vi "HEWH RLT PRAT.vi"() -> ()   [LabVIEW 2023] (continued)
        n1520 = call-poly "Enqueue Message.vi"("Priority Message? (F)"=TRUE, "Message"="Reset_Totalizer_UI", "Message Queue"=w3738) -> ("error out"=w3740:errorcluster, "dup Message Queue"=w3739:refnum<queue>)  [unwired: 7 in]
      }
      event "Reset Power Analyzer", "Start/Pause test": Value Change {
        n1521 = event-data() -> ()  [unwired: 1 in, 1 out]
        n1522 = call-poly "Enqueue Message.vi"("Priority Message? (F)"=TRUE, "Message"="Reset_PowerAnalyzer_UI", "Message Queue"=w3743) -> ("error out"=w3745:errorcluster, "dup Message Queue"=w3744:refnum<queue>)  [unwired: 7 in]
      }
      event "Manual Heating Value": Value Change {
        n1523 = event-data() -> ("NewVal"=w3748:bool)  [unwired: 1 in, 2 out]
        n1524 = call-poly "Enqueue Message.vi"("Priority Message? (F)"=TRUE, "Message Data"=w3748, "Message"="Manual_Heating_Value_UI", "Message Queue"=w3749) -> ("error out"=w3751:errorcluster, "dup Message Queue"=w3750:refnum<queue>)  [unwired: 6 in]
      }
      event "HHV-LP-Manual": Value Change {
        n1525 = event-data() -> ("NewVal"=w3754:sgl)  [unwired: 1 in, 2 out]
        n1526 = call-poly "Enqueue Message.vi"("Priority Message? (F)"=TRUE, "Message Data"=w3754, "Message"="Heating_Value_Adjust_LP_UI", "Message Queue"=w3755) -> ("error out"=w3757:errorcluster, "dup Message Queue"=w3756:refnum<queue>)  [unwired: 6 in]
      }
      event "HHV-NG-Manual": Value Change {
        n1527 = event-data() -> ("NewVal"=w3760:sgl)  [unwired: 1 in, 2 out]
        n1528 = call-poly "Enqueue Message.vi"("Priority Message? (F)"=TRUE, "Message Data"=w3760, "Message"="Heating_Value_Adjust_NG_UI", "Message Queue"=w3761) -> ("error out"=w3763:errorcluster, "dup Message Queue"=w3762:refnum<queue>)  [unwired: 6 in]
      }
      event "Update Vesta Temp": Value Change {
        n1529 = event-data() -> ()  [unwired: 1 in, 3 out]
        n1530 = call-poly "Enqueue Message.vi"("Priority Message? (F)"=TRUE, "Message Data"="Temperature Parameters", "Message"="PUT_Vesta_Temp_UI", "Message Queue"=w3768) -> ("dup Message Queue"=w3767:refnum<queue>)  [unwired: 6 in, 1 out]
      }
      event "Update Enviracom Status": Value Change {
        n1531 = event-data() -> ()  [unwired: 1 in, 1 out]
        n1532 = case shown="\"Burner OFF\", Default" "Burner Status" {
          tunnel: [FALSE TRUE] -> w3771
          frame "Burner OFF", Default {
          }
          frame "Burner ON" {
          }
        }
        n1533 = call-poly "Enqueue Message.vi"("Priority Message? (F)"=TRUE, "Message Data"=w3771, "Message"="PUT_EnviraCom_Temp_UI", "Message Queue"=w3775) -> ("error out"=w3773:errorcluster, "dup Message Queue"=w3774:refnum<queue>)  [unwired: 6 in]
      }
      event "Vesta COM Port": Value Change {
        n1534 = event-data() -> ("NewVal"=w3781:refnum<visa-resource-name>)  [unwired: 1 in]
        n1535 = property class="Instr"(reference=w3781) -> ("Rsrc Name"=w3780:string)  [unwired: 1 in, 2 out]
        n1536 = call-poly "Enqueue Message.vi"("Priority Message? (F)"=TRUE, "Message Data"=w3780, "Message"="Set_Vesta_VISA_Name_UI", "Message Queue"=w3784) -> ("error out"=w3782:errorcluster, "dup Message Queue"=w3783:refnum<queue>)  [unwired: 6 in]
      }
      event "Ultramat  COM Port": Value Change {
        n1537 = event-data() -> ("NewVal"=w3788:refnum<visa-resource-name>)  [unwired: 1 in]
        n1538 = property class="Serial Instr"(reference=w3788) -> ("Rsrc Name"=w3787:string)  [unwired: 1 in, 2 out]
        n1539 = call-poly "Enqueue Message.vi"("Priority Message? (F)"=TRUE, "Message Data"=w3787, "Message"="Set_Ultramat_VISA_Name_UI", "Message Queue"=w3791) -> ("error out"=w3789:errorcluster, "dup Message Queue"=w3790:refnum<queue>)  [unwired: 6 in]
      }
      event "MW100 COM Port": Value Change {
        n1540 = event-data() -> ("NewVal"=w3795:refnum<visa-resource-name>)  [unwired: 1 in]
        n1541 = property class="Instr"(reference=w3795) -> ("Rsrc Name"=w3794:string)  [unwired: 1 in, 2 out]
        n1542 = call-poly "Enqueue Message.vi"("Priority Message? (F)"=TRUE, "Message Data"=w3794, "Message"="Set_MW100_VISA_Name_UI", "Message Queue"=w3798) -> ("error out"=w3796:errorcluster, "dup Message Queue"=w3797:refnum<queue>)  [unwired: 6 in]
      }
      event "Agilent COM Port": Value Change {
        n1543 = event-data() -> ("NewVal"=w3802:refnum<visa-resource-name>)  [unwired: 1 in]
        n1544 = property class="Instr"(reference=w3802) -> ("Rsrc Name"=w3801:string)  [unwired: 1 in, 2 out]
        n1545 = call-poly "Enqueue Message.vi"("Priority Message? (F)"=TRUE, "Message Data"=w3801, "Message"="Set_Agilent_VISA_Name_UI", "Message Queue"=w3805) -> ("error out"=w3803:errorcluster, "dup Message Queue"=w3804:refnum<queue>)  [unwired: 6 in]
      }
      event "Alicat COM Port": Value Change {
        n1546 = event-data() -> ("NewVal"=w3809:refnum<visa-resource-name>)  [unwired: 1 in]
        n1547 = property class="Instr"(reference=w3809) -> ("Rsrc Name"=w3808:string)  [unwired: 1 in, 2 out]
        n1548 = call-poly "Enqueue Message.vi"("Priority Message? (F)"=TRUE, "Message Data"=w3808, "Message"="Set_Alicat_VISA_Name_UI", "Message Queue"=w3812) -> ("error out"=w3810:errorcluster, "dup Message Queue"=w3811:refnum<queue>)  [unwired: 6 in]
      }
      event "Ritter COM Port": Value Change {
        n1549 = event-data() -> ("NewVal"=w3816:refnum<visa-resource-name>)  [unwired: 1 in]
        n1550 = property class="Instr"(reference=w3816) -> ("Rsrc Name"=w3815:string)  [unwired: 1 in, 2 out]
        n1551 = call-poly "Enqueue Message.vi"("Priority Message? (F)"=TRUE, "Message Data"=w3815, "Message"="Set_Ritter_VISA_Name_UI", "Message Queue"=w3819) -> ("error out"=w3817:errorcluster, "dup Message Queue"=w3818:refnum<queue>)  [unwired: 6 in]
      }
      event "Heise Barometer COM Port": Value Change {
        n1552 = event-data() -> ("NewVal"=w3823:refnum<visa-resource-name>)  [unwired: 1 in]
        n1553 = property class="Instr"(reference=w3823) -> ("Rsrc Name"=w3822:string)  [unwired: 1 in, 2 out]
        n1554 = call-poly "Enqueue Message.vi"("Priority Message? (F)"=TRUE, "Message Data"=w3822, "Message"="Set_Heise_VISA_Name_UI", "Message Queue"=w3826) -> ("error out"=w3824:errorcluster, "dup Message Queue"=w3825:refnum<queue>)  [unwired: 6 in]
      }
      event "WT300 COM Port": Value Change {
        n1555 = event-data() -> ("NewVal"=w3830:refnum<visa-resource-name>)  [unwired: 1 in]
        n1556 = property class="Instr"(reference=w3830) -> ("Rsrc Name"=w3829:string)  [unwired: 1 in, 2 out]
        n1557 = call-poly "Enqueue Message.vi"("Priority Message? (F)"=TRUE, "Message Data"=w3829, "Message"="Set_WT300_VISA_Name_UI", "Message Queue"=w3833) -> ("error out"=w3831:errorcluster, "dup Message Queue"=w3832:refnum<queue>)  [unwired: 6 in]
      }
      event "Laurel IP Address": Value Change {
        n1558 = event-data() -> ("NewVal"=w3836:string)  [unwired: 1 in]
        n1559 = call-poly "Enqueue Message.vi"("Priority Message? (F)"=TRUE, "Message Data"=w3836, "Message"="Set_Laurel_IP_Name_UI", "Message Queue"=w3839) -> ("error out"=w3837:errorcluster, "dup Message Queue"=w3838:refnum<queue>)  [unwired: 6 in]
      }
      event "Emerson IP Address": Value Change {
        n1560 = event-data() -> ("NewVal"=w3842:string)  [unwired: 1 in]
        n1561 = call-poly "Enqueue Message.vi"("Priority Message? (F)"=TRUE, "Message Data"=w3842, "Message"="Set_Emerson_IP_Name_UI", "Message Queue"=w3845) -> ("error out"=w3843:errorcluster, "dup Message Queue"=w3844:refnum<queue>)  [unwired: 6 in]
      }
      event "NG Inficon IP Address": Value Change {
        n1562 = event-data() -> ("NewVal"=w3848:string)  [unwired: 1 in]
        n1563 = call-poly "Enqueue Message.vi"("Priority Message? (F)"=TRUE, "Message Data"=w3848, "Message"="Set_NG_Inficon_IP_Name_UI", "Message Queue"=w3851) -> ("error out"=w3849:errorcluster, "dup Message Queue"=w3850:refnum<queue>)  [unwired: 6 in]
      }
      event "LP Inficon IP Address": Value Change {
        n1564 = event-data() -> ("NewVal"=w3854:string)  [unwired: 1 in]
        n1565 = call-poly "Enqueue Message.vi"("Priority Message? (F)"=TRUE, "Message Data"=w3854, "Message"="Set_LP_Inficon_IP_Name_UI", "Message Queue"=w3857) -> ("error out"=w3855:errorcluster, "dup Message Queue"=w3856:refnum<queue>)  [unwired: 6 in]
      }
      event "Viasala IP Address": Value Change {
        n1566 = event-data() -> ("NewVal"=w3860:string)  [unwired: 1 in]
        n1567 = call-poly "Enqueue Message.vi"("Priority Message? (F)"=TRUE, "Message Data"=w3860, "Message"="Set_Viasala_IP_Name_UI", "Message Queue"=w3863) -> ("error out"=w3861:errorcluster, "dup Message Queue"=w3862:refnum<queue>)  [unwired: 6 in]
      }
      event "Tenney IP Address": Value Change {
        n1568 = event-data() -> ("NewVal"=w3866:string)  [unwired: 1 in]
        n1569 = call-poly "Enqueue Message.vi"("Priority Message? (F)"=TRUE, "Message Data"=w3866, "Message"="Set_Tenney_IP_Name_UI", "Message Queue"=w3869) -> ("error out"=w3867:errorcluster, "dup Message Queue"=w3868:refnum<queue>)  [unwired: 6 in]
      }
      event Value Change {
        n1570 = event-data() -> ("NewVal"=w3872:T50)  [unwired: 1 in]
        n1571 = call-poly "Enqueue Message.vi"("Priority Message? (F)"=TRUE, "Message Data"=w3872, "Message"="Set_Agilent_Station_UI", "Message Queue"=w3875) -> ("error out"=w3873:errorcluster, "dup Message Queue"=w3874:refnum<queue>)  [unwired: 6 in]
      }
      event Value Change {
        n1572 = event-data() -> ("NewVal"=w3879:T49)  [unwired: 1 in]
        n1573 = call-poly "Enqueue Message.vi"("Priority Message? (F)"=TRUE, "Message Data"=w3879, "Message"="GEA3_StationA_Board_ID_UI", "Message Queue"=w3880) -> ("error out"=w3881:errorcluster, "dup Message Queue"=w3878:refnum<queue>)  [unwired: 6 in]
      }
      event Value Change {
        n1574 = event-data() -> ("NewVal"=w3885:T49)  [unwired: 1 in]
        n1575 = call-poly "Enqueue Message.vi"("Priority Message? (F)"=TRUE, "Message Data"=w3885, "Message"="GEA3_StationB_Board_ID_UI", "Message Queue"=w3886) -> ("error out"=w3887:errorcluster, "dup Message Queue"=w3884:refnum<queue>)  [unwired: 6 in]
      }
      event Value Change {
        n1576 = event-data() -> ("NewVal"=w3891:T49)  [unwired: 1 in]
        n1577 = call-poly "Enqueue Message.vi"("Priority Message? (F)"=TRUE, "Message Data"=w3891, "Message"="GEA3_StationC_Board_ID_UI", "Message Queue"=w3892) -> ("error out"=w3893:errorcluster, "dup Message Queue"=w3890:refnum<queue>)  [unwired: 6 in]
      }
      event Value Change {
        n1578 = event-data() -> ("NewVal"=w3897:T49)  [unwired: 1 in]
        n1579 = call-poly "Enqueue Message.vi"("Priority Message? (F)"=TRUE, "Message Data"=w3897, "Message"="GEA3_StationD_Board_ID_UI", "Message Queue"=w3898) -> ("error out"=w3899:errorcluster, "dup Message Queue"=w3896:refnum<queue>)  [unwired: 6 in]
      }
      event "Enviracom COM Port": Value Change {
        n1580 = event-data() -> ("NewVal"=w3903:refnum<visa-resource-name>)  [unwired: 1 in]
        n1581 = property class="Instr"(reference=w3903) -> ("Rsrc Name"=w3902:string)  [unwired: 1 in, 2 out]
        n1582 = call-poly "Enqueue Message.vi"("Priority Message? (F)"=TRUE, "Message Data"=w3902, "Message"="Set_Envira_VISA_Name_UI", "Message Queue"=w3906) -> ("error out"=w3904:errorcluster, "dup Message Queue"=w3905:refnum<queue>)  [unwired: 6 in]
      }
    }
    n1583 = call "Tenney Error Handler - Event Handling Loop.vi"("error in (no error)"=w3410, "Message Queue"=w3408) -> ("dup error in"=w3407:errorcluster)  [unwired: 8 in, 1 out]
  }
  n1584 = while {
    tunnel: w59 -> [w3937]
    shift-right: [w3943] -> _
    shift-left: T67 {"Timer Data"={"Station A-Timer"=[], "Station B-Timer"=[], "Station C-Timer"=[], "Station D-Timer"=[], "Timer A"=0.0, "Timer B"=0.0, "Timer C"=0.0, "Timer D"=0.0, "TimerA (String)"="", "TimerB (String)"="", "TimerC (String)"="", "TimerD (String)"="", "TimerA (H:M:S)"="", "TimerB (H:M:S)"="", "TimerC (H:M:S)"="", "TimerD (H:M:S)"=""}, "Tenney Data"={"Temperature Setpoint"=0.0, "Temperature Process Variable"=0.0, "Humidity Setpoint"=0.0, "Humidity Process Variable"=0.0, "Frequency Setpoint"=0.0, "Frequency Process Variable"=0.0, "Chamber Status (ON/OFF)"=""}, "Viasala Data Output"={"Temperature Probe 1"=0.0, "Humidity Probe 1"=0.0, "Temperature Probe 2"=0.0, "Humidity Probe 2"=0.0}, "Alicat Data"={"Data Cluster"={"Absolute Pressure"=0.0, "Gauge/Diff. Pressure"=0.0, "Barometric Pressure"=0.0, "Temperature"=0.0, "Volumetric Flow"=0.0, "Mass Flow"=0.0, "Setpoint"=0.0, "Valve Drive"=0.0, "Totalizer"=0.0, "[hr]"=0.0, "[min]"=0.0, "[sec]"=0.0, "Totalizer Average Flow"=0.0, "Totalizer Peak Flow"=0.0, "Gas selected"=""}, "Units of Measure Input"={"Abs. Pressure"="", "Gauge/Diff. Press."="", "Barometric Press."="", "Temperature"="", "Volume"="", "Mass"="", "Setpoint"="", "Valve Drive"="", "Totalizer"="", "Tot. Timer"="", "Tot. Avg. Flow"="", "Tot. Peak Flow"=""}, "Header Array"=[]}, "Inficon Data"={"Gross Heating Value, Vol (Real, Dry)"=0.0, "Nitrogen Component Normalized Mole % (Dry)"=0.0, "Methane Component Normalized Mole % (Dry)"=0.0, "Carbon Dioxide Component Normalized Mole % (Dry)"=0.0, "Ethane Component Normalized Mole % (Dry)"=0.0, "Propane Component Normalized Mole % (Dry)"=0.0, "i-Pentane Component Normalized Mole % (Dry)"=0.0, "i-Butane Component Normalized Mole % (Dry)"=0.0, "n-Butane Component Normalized Mole % (Dry)"=0.0, "n-Pentane Component Normalized Mole % (Dry)"=0.0, "Hexane Component Normalized Mole % (Dry)"=0.0, "Heptane Component Normalized Mole % (Dry)"=0.0, "Gross Wobbe Index, Real(Dry)"=0.0, "Relative Density, Real(Dry)"=0.0, "Propylene Component Normalized Mole % (Dry)"=0.0, "C4 Olefins Component Normalized Mole % (Dry)"=0.0, "Water Component Normalized Mole % (Dry)"=0.0, "Gross Heating Value, Vol (Real, Sat)"=0.0, "Natural Gas Data"=[], "Propane Data"=[]}, "Inficon Data LP"={"Gross Heating Value, Vol (Real, Dry)"=0.0, "Nitrogen Component Normalized Mole % (Dry)"=0.0, "Methane Component Normalized Mole % (Dry)"=0.0, "Carbon Dioxide Component Normalized Mole % (Dry)"=0.0, "Ethane Component Normalized Mole % (Dry)"=0.0, "Propane Component Normalized Mole % (Dry)"=0.0, "i-Pentane Component Normalized Mole % (Dry)"=0.0, "i-Butane Component Normalized Mole % (Dry)"=0.0, "n-Butane Component Normalized Mole % (Dry)"=0.0, "n-Pentane Component Normalized Mole % (Dry)"=0.0, "Hexane Component Normalized Mole % (Dry)"=0.0, "Heptane Component Normalized Mole % (Dry)"=0.0, "Gross Wobbe Index, Real(Dry)"=0.0, "Relative Density, Real(Dry)"=0.0, "Propylene Component Normalized Mole % (Dry)"=0.0, "C4 Olefins Component Normalized Mole % (Dry)"=0.0, "Water Component Normalized Mole % (Dry)"=0.0, "Gross Heating Value, Vol (Real, Sat)"=0.0, "Natural Gas Data"=[], "Propane Data"=[]}, "Ultramat 23 Data"=[], "Ritter Data"={"Gas Flow Rate (L/hr)-Uncorrected"=0.0, "Totalized Flow (L)--Uncorrected"=0.0, "Gas Flow Rate (cuft/hr)-Uncorrected"=0.0, "Totalized Flow (cuft)-Uncorrected"=0.0, "Gas Temperature (F)"=0.0, "Gas Pressure (in WC)"=0.0, "Heise Barometric Pressure (inHG)"=0.0, "STP Correction Factor"=0.0, "Temp Correction Factor"=0.0, "Pressure Correction Factor"=0.0, "Water Vapor Pressure"=0.0, "Gas Flow Rate (cuft/hr)-Corrected"=0.0, "Totalized Flow (cuft)-Corrected"=0.0, "Gas BTU"=0.0, "Gas BTU/hr"=0.0, "Gas Flow Rate (cuft/hr)-Uncorrected-Raw"=0.0}, "Heise Data"=0.0, "Emerson Data"={"Mass Flow Rate (Scaled Integer)"=0, "Density (Scaled Integer)"=0, "Temperature (Scaled Integer)"=0, "Volume Flow Rate (Scaled Integer)"=0, "Totalizer 1 (Scaled Integer)"=0, "Totalizer 2 (Scaled Integer)"=0, "Transmitter Software Rev"=0, "Flow Direction"="", "Mass Flow Units"="", "Density Units"="", "Temperature Units"="", "Volume Flow Units"="", "Pressure Units"="", "Mass Total Units"="", "Volume Total Units"="", "Inventory 1 (Scaled Integer)"=0, "Inventory 2 (Scaled Integer)"=0, "Mass Flow Rate"=0.0, "Density"=0.0, "Temperature"=0.0, "Volume Flow Rate"=0.0, "Pressure (Scaled Integer)"=0, "Current Value Totalizer 1 (Pounds per draw)"=0.0, "Current Value Totalizer 2 (Gallons per draw)"=0.0, "Current Value Inventory 1 (Pounds Total)"=0.0, "Current Value Inventory 2 (Gallons Total)"=0.0, "Drive Gain"=0.0, "Raw Tube Frequency (Hz)"=0.0, "Dynamic Viscosity (Centipoise)"=0.0, "Kinematic Viscosity (Centistokes)"=0.0, "Hot Gallons (Calculated Gallons)"=0.0, "Hot Flow Rate (Calculated GPM)"=0.0, "Hot Gallons Inventory (Gallons)"=0.0, "Hot Flow Rate (Laurel)"=0.0, "Hot Gallons (Laurel)"=0.0}, "Laurel Meter Data"={"Flow Rate (GPM)"=0.0, "Totalized Flow (Gallons)"=0.0}, "WT300 Data"={"Current (A):Element 1"=0.0, "Current (A):Element 2"=0.0, "Power (W):Sigma"=0.0, "Watt Hours (Wh):Sigma"=0.0, "Voltage (V):Element 2"=0.0, "Voltage (V):Element 1"=0.0, "Current Crest Factor:Element 1"=0.0, "Current Crest Factor:Element 2"=0.0, "Voltage Harmonic (%):Element 1"=0.0, "Voltage Harmonic (%):Element 2"=0.0, "Voltage Crest Factor:Element 1"=0.0, "Voltage Crest Factor:Element 2"=0.0, "Time:Element 1"=0.0, "Frequency (Hz):Element 1"=0.0, "Apparent Power (VA):Element 1"=0.0, "Apparent Power (VA):Element 2"=0.0, "Power Factor:Element 1"=0.0, "Power Factor:Element 2"=0.0, "Max Watt Hours"=0.0, "Voltage (V):Element 2 Avg"=0.0, "Voltage (V):Element 1 Avg"=0.0}, "Agilent Data"={"Location 11 (Channel 111)"=0.0, "Location 12 (Channel 112)"=0.0, "Location 13 (Channel 113)"=0.0, "Location 14 (Channel 114)"=0.0, "Location 15 (Channel 115)"=0.0, "Location 16 (Channel 116)"=0.0, "Location 17 (Channel 109)"=0.0, "Location 18 (Channel 110)"=0.0, "Location 19 (Channel 201)"=0.0, "Location 20 (Channel 202)"=0.0, "Location 21 (Channel 203)"=0.0, "Location 22 (Channel 204)"=0.0, "Location 23 (Channel 205)"=0.0, "Location 24 (Channel 206)"=0.0, "Location 25 (Channel 207)"=0.0, "Location 26 (Channel 208)"=0.0, "Location 27 (Channel 209)"=0.0, "Location 28 (Channel 210)"=0.0, "Location 29 (Channel 211)"=0.0, "Location 30 (Channel 212)"=0.0, "Location 31 (Channel 213)"=0.0, "Location 32 (Channel 214)"=0.0, "Location 33 (Channel 215)"=0.0, "Location 34 (Channel 216)"=0.0, "Location 35 (Channel 107)"=0.0, "Location 36 (Channel 108)"=0.0, "Location 37 (Channel 301)"=0.0, "Location 38 (Channel 302)"=0.0, "Location 39 (Channel 303)"=0.0, "Location 40 (Channel 304)"=0.0, "Location 41 (Channel 305)"=0.0, "Location 42 (Channel 306)"=0.0, "Location 43 (Channel 307)"=0.0, "Location 44 (Channel 308)"=0.0, "Location 45 (Channel 309)"=0.0, "Location 46 (Channel 310)"=0.0, "Location 47 (Channel 311)"=0.0, "Location 48 (Channel 312)"=0.0, "Location 49 (Channel 313)"=0.0, "Location 50 (Channel 314)"=0.0, "Location 51 (Channel 315)"=0.0, "Location 52 (Channel 316)"=0.0, "Location 53 (Channel 105)"=0.0, "Location 54 (Channel 106)"=0.0}, "GEA Data - Station A"={"ERD Data Input"={"Mixing Valve"={"T7 Temp (°F) - (0x40B9)"=0.0, "MixValveAbsoluteStepPosition - (0x400B)"=0, "Flow State - (0X4069)"=0, "T6 Temp (°F) - (0x406E)"=0.0}, "Standard ERDs"={"User UI Mode (0X4020)"="", "User Setpoint (0x4024)"=0, "Compressor (0x4068)"=FALSE, "Lower Element (0x4068)"=FALSE, "Upper Element (0x4068)"=FALSE, "Fan (0x4068)"=FALSE, "T1 Temp Lower Tank (°F) - (0x405F)"=0.0, "T2 Temp Upper Tank (°F) - (0x4060)"=0.0, "Line Voltage (0x4066)"=0, "MeasuredCurrent (0x4065)"=0.0, "Tank Setpoint (°F) - (0x4026)"=0, "Depletion - (0x40CB)"=0, "Personality - (0x0035)"=0}, "Heat Pump"={"EEV Position - (0X4067)"=0, "T3A TEMP EVAP IN (°F) - (0x4061)"=0.0, "T3B TEMP EVAP OUT (°F) -(0x4062)"=0.0, "T4 TEMP COMP DISCHARGE (°F) - (0x4063)"=0.0, "T5 TEMP AMBIENT (°F)- (0x4064)"=0.0, "Condensate Sensor - (0x40BC)"=0, "Fan (RPM) - (0xF073)"=0, "PWM (%) - (0xF056)"=0, "Compressor Speed (RPM) - (0xF093)"=0, "Compressor Target (RPM) - (0xF081)"=0, "Compressor Power (W) - (0xF092)"=0, "CPU Temperature (°F) - (0x40BA)"=0.0, "Board Temperature (°F) - (0x40BB)"=0.0}, "Inverter"={"Inverter IGBT Temp (°C) - (0xF280)"=0.0, "Inverter Chip Temp (°C) - (0xF284)"=0.0}}, "ERD Data"=[]}, "GEA Data - Station B"={"ERD Data Input"={"Mixing Valve"={"T7 Temp (°F) - (0x40B9)"=0.0, "MixValveAbsoluteStepPosition - (0x400B)"=0, "Flow State - (0X4069)"=0, "T6 Temp (°F) - (0x406E)"=0.0}, "Standard ERDs"={"User UI Mode (0X4020)"="", "User Setpoint (0x4024)"=0, "Compressor (0x4068)"=FALSE, "Lower Element (0x4068)"=FALSE, "Upper Element (0x4068)"=FALSE, "Fan (0x4068)"=FALSE, "T1 Temp Lower Tank (°F) - (0x405F)"=0.0, "T2 Temp Upper Tank (°F) - (0x4060)"=0.0, "Line Voltage (0x4066)"=0, "MeasuredCurrent (0x4065)"=0.0, "Tank Setpoint (°F) - (0x4026)"=0, "Depletion - (0x40CB)"=0, "Personality - (0x0035)"=0}, "Heat Pump"={"EEV Position - (0X4067)"=0, "T3A TEMP EVAP IN (°F) - (0x4061)"=0.0, "T3B TEMP EVAP OUT (°F) -(0x4062)"=0.0, "T4 TEMP COMP DISCHARGE (°F) - (0x4063)"=0.0, "T5 TEMP AMBIENT (°F)- (0x4064)"=0.0, "Condensate Sensor - (0x40BC)"=0, "Fan (RPM) - (0xF073)"=0, "PWM (%) - (0xF056)"=0, "Compressor Speed (RPM) - (0xF093)"=0, "Compressor Target (RPM) - (0xF081)"=0, "Compressor Power (W) - (0xF092)"=0, "CPU Temperature (°F) - (0x40BA)"=0.0, "Board Temperature (°F) - (0x40BB)"=0.0}, "Inverter"={"Inverter IGBT Temp (°C) - (0xF280)"=0.0, "Inverter Chip Temp (°C) - (0xF284)"=0.0}}, "ERD Data"=[]}, "GEA Data - Station C"={"ERD Data Input"={"Mixing Valve"={"T7 Temp (°F) - (0x40B9)"=0.0, "MixValveAbsoluteStepPosition - (0x400B)"=0, "Flow State - (0X4069)"=0, "T6 Temp (°F) - (0x406E)"=0.0}, "Standard ERDs"={"User UI Mode (0X4020)"="", "User Setpoint (0x4024)"=0, "Compressor (0x4068)"=FALSE, "Lower Element (0x4068)"=FALSE, "Upper Element (0x4068)"=FALSE, "Fan (0x4068)"=FALSE, "T1 Temp Lower Tank (°F) - (0x405F)"=0.0, "T2 Temp Upper Tank (°F) - (0x4060)"=0.0, "Line Voltage (0x4066)"=0, "MeasuredCurrent (0x4065)"=0.0, "Tank Setpoint (°F) - (0x4026)"=0, "Depletion - (0x40CB)"=0, "Personality - (0x0035)"=0}, "Heat Pump"={"EEV Position - (0X4067)"=0, "T3A TEMP EVAP IN (°F) - (0x4061)"=0.0, "T3B TEMP EVAP OUT (°F) -(0x4062)"=0.0, "T4 TEMP COMP DISCHARGE (°F) - (0x4063)"=0.0, "T5 TEMP AMBIENT (°F)- (0x4064)"=0.0, "Condensate Sensor - (0x40BC)"=0, "Fan (RPM) - (0xF073)"=0, "PWM (%) - (0xF056)"=0, "Compressor Speed (RPM) - (0xF093)"=0, "Compressor Target (RPM) - (0xF081)"=0, "Compressor Power (W) - (0xF092)"=0, "CPU Temperature (°F) - (0x40BA)"=0.0, "Board Temperature (°F) - (0x40BB)"=0.0}, "Inverter"={"Inverter IGBT Temp (°C) - (0xF280)"=0.0, "Inverter Chip Temp (°C) - (0xF284)"=0.0}}, "ERD Data"=[]}, "GEA Data - Station D"={"ERD Data Input"={"Mixing Valve"={"T7 Temp (°F) - (0x40B9)"=0.0, "MixValveAbsoluteStepPosition - (0x400B)"=0, "Flow State - (0X4069)"=0, "T6 Temp (°F) - (0x406E)"=0.0}, "Standard ERDs"={"User UI Mode (0X4020)"="", "User Setpoint (0x4024)"=0, "Compressor (0x4068)"=FALSE, "Lower Element (0x4068)"=FALSE, "Upper Element (0x4068)"=FALSE, "Fan (0x4068)"=FALSE, "T1 Temp Lower Tank (°F) - (0x405F)"=0.0, "T2 Temp Upper Tank (°F) - (0x4060)"=0.0, "Line Voltage (0x4066)"=0, "MeasuredCurrent (0x4065)"=0.0, "Tank Setpoint (°F) - (0x4026)"=0, "Depletion - (0x40CB)"=0, "Personality - (0x0035)"=0}, "Heat Pump"={"EEV Position - (0X4067)"=0, "T3A TEMP EVAP IN (°F) - (0x4061)"=0.0, "T3B TEMP EVAP OUT (°F) -(0x4062)"=0.0, "T4 TEMP COMP DISCHARGE (°F) - (0x4063)"=0.0, "T5 TEMP AMBIENT (°F)- (0x4064)"=0.0, "Condensate Sensor - (0x40BC)"=0, "Fan (RPM) - (0xF073)"=0, "PWM (%) - (0xF056)"=0, "Compressor Speed (RPM) - (0xF093)"=0, "Compressor Target (RPM) - (0xF081)"=0, "Compressor Power (W) - (0xF092)"=0, "CPU Temperature (°F) - (0x40BA)"=0.0, "Board Temperature (°F) - (0x40BB)"=0.0}, "Inverter"={"Inverter IGBT Temp (°C) - (0xF280)"=0.0, "Inverter Chip Temp (°C) - (0xF284)"=0.0}}, "ERD Data"=[]}, "MW100 Data"={"TC1-Channel 021"=0.0, "TC2-Channel 022"=0.0, "TC3-Channel 023"=0.0, "TC4-Channel 024"=0.0, "TC5-Channel 025"=0.0, "TC6-Channel 026"=0.0, "TC7-Channel 017"=0.0, "TC8-Channel 028"=0.0, "TC9-Channel 029"=0.0, "TC10-Channel 030"=0.0, "TC Tree Average"=0.0, "TC DWN- Channel 027"=0.0, "RTDin-Channel 031"=0.0, "RTDout-Channel 032"=0.0, "RTDamb-Channel 033"=0.0, "PSI1-Channel 011"=0.0, "PSI2-Channel 012"=0.0, "PSI3-Channel 013"=0.0, "PSI4-Channel 014"=0.0, "UE State-Channel 015"=0.0, "LE State-Channel 016"=0.0, "Module 4 Relay Status Output"={"INTELLIFAUCET TEMP(T)/FLOW(F) (CH 041)"=FALSE, "INTELLIFAUCET READY (CH 042)"=FALSE, "INTELLIFAUCET START (CH 043)"=FALSE, "INTELLIFAUCET STOP (CH 044)"=FALSE, "MAIN POWER RELAY (CH 047)"=FALSE, "NOT USED (CH 045)"=FALSE, "NOT USED (CH 046)"=FALSE, "PURGE VALVE RELAY (CH 048)"=FALSE, "OUTLET VALVE RELAY (CH 049)"=FALSE, "INLET VALVE RELAY (CH 050)"=FALSE, "Intellifaucet (% Open)"=0.0, "Proportioning Valve (%Open)"=0.0, "Intellifaucet Temp Setpoint (F)"=0.0}}, "Vesta Data Output"={"Temp_W_Raw_U"=0, "Temp_W_Raw_L"=0, "Temperature Water (F)"=0.0, "Temperature Water Compensated (F)"=0.0, "Temperature Ambient (F)"=0.0, "Setpoint Location (F)"=0.0, "Heat Request"="", "Fault Ram"="", "PWM DCDC Value"=0, "Pilot Voltage (mV)"=0.0, "Setpoint Actual (F)"=0.0, "Differential Actual (F)"=0.0, "Setpoint User (F)"=0.0, "Differential User (F)"=0.0, "Termperature FIltered -TCO (F)"=0.0, "Temp_C_Raw_1 - Sensor Voltage"="", "Temp_C_Raw_2 - Sensor Voltage"="", "Chamber Sensor Temperature (F)"=0.0, "LDO Base Temperature (F)"=0.0, "LDO Timer (sec)"=0, "Disabled (0)"=FALSE, "Warming (1)"=FALSE, "Heating (2)"=FALSE, "Cooling Data Write (3)"=FALSE, "Cooling (4)"=FALSE, "Data Read (5)"=FALSE, "N/A"=FALSE, "Temperature Trip (7)"=FALSE, "Burner"=FALSE}} ("Data Cluster") -> [w3944]
    tunnel: w68 -> [w3941]
    tunnel: w69 -> [w3940]
    tunnel: [w3935] -> w58
    tunnel: w72 -> [w3933]
    shift-right: [w3931] -> _
    shift-left: string[] [] -> [w3932]
    tunnel: w76 -> [w3929]
    tunnel: w55 -> [w3927]
    tunnel: w49 -> [w3926]
    tunnel: w48 -> [w3925]
    tunnel: w45 -> [w3924]
    tunnel: w43 -> [w3923]
    tunnel: w40 -> [w3922]
    tunnel: w35 -> [w3921]
    tunnel: w29 -> [w3920]
    tunnel: w28 -> [w3919]
    tunnel: w27 -> [w3918]
    tunnel: w26 -> [w3917]
    tunnel: w25 -> [w3916]
    tunnel: w24 -> [w3915]
    tunnel: w23 -> [w3914]
    tunnel: w22 -> [w3913]
    tunnel: w21 -> [w3912]
    tunnel: w20 -> [w3911]
    tunnel: w19 -> [w3910]
    tunnel: w18 -> [w3909]
    stop <- w3942 stop-if-true
    # "Message Handling Loop"
    n1585 = call "Dequeue Message.vi"("error in (no error)"=w3940, "Message Queue"=w3937) -> ("error out"=w3939:errorcluster, "Message Data"=w3938:variant, "Message"=w3930:string, "dup Message Queue"=w3936:refnum<queue>)  [unwired: 6 in]
    n1586 = case "Message Cases" shown="\"Process_Data\"" w3930 {
      selector: w3930 -> [_ w3952 _ _ _ _ _ _ _ _ _ _ _ _ _ _ _ _ _ _ _ _ _ _ _ _ _ _ _ _ _ _ _ _ _ _ _ _ _ _ _ _ _ _ _ _ _ _ _ _ _ _ _ _ _ _ _ _ _ _ _ _ _ _ _ _ _ _ _ _ _ _ _ _ _ _ _ _ _ _ _ _ _ _ _ _ _ _ _ _ _ _ _ _ _ _ _ _ _ _ _ _ _ _ _ _ _ _ _ _ _ _ _ _ _ _ _ _ _ _ _ _ _ _ _ _ _ _ _ _]
      tunnel: w3936 -> [_ _ w3970 _ w3996 _ _ _ _ _ _ _ w4030 _ _ _ _ _ _ _ _ _ _ _ _ _ _ _ _ _ _ _ _ _ _ _ _ w4205 _ _ _ _ _ _ _ _ w4281 _ _ _ _ _ _ _ _ _ _ _ _ w4386 _ _ w4409 _ _ w4432 _ _ w4455 _ _ w4478 _ _ _ _ _ _ _ _ _ _ _ _ _ _ w4606 _ _ _ w4638 _ _ w4661 _ _ _ _ w4700 _ _ _ w4729 _ _ _ _ w4773 _ _ _ w4806 _ _ _ w4841 _ _ _ _ _ w4884 _ _ _ w4915 _ _ _ w4948]
      tunnel: w3939 -> [w3951 _ w3969 w3977 w3990 w3999 w4003 w4004 w4011 w4017 w4023 w4029 w4039 w4040 w4048 w4058 w4065 w4072 w4079 w4086 w4093 w4100 w4107 w4114 w4121 w4128 w4135 w4142 w4149 w4156 w4163 w4170 w4176 w4182 w4189 w4196 w4203 w4213 w4215 w4223 w4231 w4243 w4251 w4259 w4266 w4274 w4290 w4292 w4300 w4306 w4314 w4322 w4330 w4338 w4345 w4353 w4361 w4369 w4379 w4395 w4397 w4405 w4418 w4420 w4428 w4441 w4443 w4451 w4464 w4466 w4474 w4487 w4489 w4492 w4505 w4517 w4529 w4541 w4559 w4560 w4572 w4579 w4586 w4588 w4596 w4605 w4615 w4617 w4625 w4637 w4647 w4649 w4657 w4670 w4672 w4680 w4689 w4699 w4709 w4711 w4719 w4724 w4738 w4740 w4748 w4757 w4769 w4782 w4784 w4792 w4802 w4815 w4817 w4825 w4835 w4848 w4850 w4858 w4868 w4872 w4880 w4893 w4895 w4903 w4909 w4924 w4926 w4934 w4944 w4957]
      tunnel: [w3949 w3953 w3966 w3971 w3993 w3997 w4002 w4004 w4007 w4013 w4019 w4025 w4031 w4040 w4045 w4054 w4061 w4068 w4075 w4082 w4089 w4096 w4103 w4110 w4117 w4124 w4131 w4138 w4145 w4152 w4159 w4166 w4172 w4178 w4185 w4192 w4199 w4214 w4215 w4220 w4236 w4244 w4252 w4260 w4271 w4279 w4291 w4292 w4297 w4310 w4318 w4326 w4334 w4342 w4349 w4357 w4365 w4373 w4376 w4396 w4397 w4402 w4419 w4420 w4425 w4442 w4443 w4448 w4465 w4466 w4471 w4488 w4489 w4491 w4502 w4515 w4527 w4539 w4552 w4560 w4572 w4579 w4586 w4588 w4593 w4600 w4616 w4617 w4622 w4634 w4648 w4649 w4654 w4671 w4672 w4677 w4685 w4691 w4710 w4711 w4716 w4725 w4739 w4740 w4745 w4760 w4765 w4783 w4784 w4789 w4798 w4816 w4817 w4822 w4831 w4849 w4850 w4854 w4864 w4872 w4877 w4894 w4895 w4900 w4913 w4925 w4926 w4931 w4941 w4958] -> w3934
      tunnel: w3944 -> [w3950 w3954 w3962 w3976 w3995 w3998 w4001 w4005 w4008 w4014 w4020 w4026 w4036 w4041 w4051 w4055 w4062 w4069 w4076 w4083 w4090 w4097 w4104 w4111 w4118 w4125 w4132 w4139 w4146 w4153 w4160 w4167 w4173 w4179 w4186 w4193 w4200 w4211 w4216 w4226 w4237 w4245 w4253 w4261 w4272 w4280 w4287 w4293 w4303 w4311 w4319 w4327 w4335 w4343 w4350 w4358 w4366 w4374 w4381 w4392 w4398 w4408 w4415 w4421 w4431 w4438 w4444 w4454 w4461 w4467 w4477 w4484 w4490 w4494 w4507 w4519 w4531 w4543 w4556 w4566 w4573 w4580 w4587 w4589 w4599 w4602 w4612 w4618 w4628 w4631 w4644 w4650 w4660 w4667 w4673 w4683 w4686 w4696 w4706 w4712 w4722 w4728 w4735 w4741 w4751 w4762 w4772 w4779 w4785 w4795 w4805 w4812 w4818 w4828 w4838 w4846 w4851 w4861 w4871 w4873 w4883 w4890 w4896 w4906 w4914 w4921 w4927 w4937 w4947 w4954]
      tunnel: [w3950 w3954 w3962 w3976 w3995 w3998 w4001 w4005 w4008 w4014 w4020 w4026 w4035 w4041 w4051 w4055 w4062 w4069 w4076 w4083 w4090 w4097 w4104 w4111 w4118 w4125 w4132 w4139 w4146 w4153 w4160 w4167 w4173 w4179 w4186 w4193 w4200 w4210 w4216 w4226 w4237 w4245 w4253 w4261 w4272 w4280 w4286 w4293 w4303 w4311 w4319 w4327 w4335 w4343 w4350 w4358 w4366 w4374 w4381 w4391 w4398 w4408 w4414 w4421 w4431 w4437 w4444 w4454 w4460 w4467 w4477 w4483 w4490 w4494 w4507 w4519 w4531 w4543 w4556 w4566 w4573 w4580 w4587 w4589 w4599 w4602 w4611 w4618 w4628 w4631 w4643 w4650 w4660 w4666 w4673 w4683 w4686 w4696 w4705 w4712 w4722 w4728 w4734 w4741 w4751 w4762 w4772 w4778 w4785 w4795 w4805 w4811 w4818 w4828 w4838 w4845 w4851 w4861 w4871 w4873 w4883 w4889 w4896 w4906 w4914 w4920 w4927 w4937 w4947 w4953] -> w3943
      tunnel: [_ _ _ _ TRUE _ _ _ _ _ _ _ _ _ _ _ _ _ _ _ _ _ _ _ _ _ _ _ _ _ _ _ _ _ _ _ _ _ _ _ _ _ _ _ _ _ _ _ _ _ _ _ _ _ _ _ _ _ _ _ _ _ _ _ _ _ _ _ _ _ _ _ _ _ _ _ _ _ _ _ _ _ _ _ _ _ _ _ _ _ _ _ _ _ _ _ _ _ _ _ _ _ _ _ _ _ _ _ _ _ _ _ _ _ _ _ _ _ _ _ _ _ _ _ _ _ _ _ _ _] -> w3942
      tunnel: w3938 -> [_ _ _ w3975 w3987 _ _ _ _ _ _ _ w4038 _ w4046 _ _ _ _ _ _ _ _ _ _ _ _ _ _ _ _ _ _ _ _ _ _ w4212 _ w4221 w4229 _ _ _ w4264 _ w4289 _ w4298 _ _ _ _ _ _ _ _ _ w4375 w4394 _ w4403 w4417 _ w4426 w4440 _ w4449 w4463 _ w4472 w4486 _ _ w4501 w4513 w4525 w4537 _ _ _ _ _ _ w4594 _ w4614 _ w4623 _ w4646 _ w4655 w4669 _ w4678 _ _ w4708 _ w4717 _ w4737 _ w4746 w4755 w4767 w4781 _ w4790 w4800 w4814 _ w4823 w4833 w4847 _ w4856 w4866 _ w4878 w4892 _ w4901 _ w4923 _ w4932 w4942 w4956]
      tunnel: w3941 -> [_ _ _ _ w3992 _ _ _ _ _ _ _ _ _ _ _ _ _ _ _ _ _ _ _ _ _ _ _ _ _ _ _ _ _ _ _ _ _ _ _ _ _ _ _ _ _ _ _ _ _ _ _ _ _ _ _ _ _ _ _ _ _ _ _ _ _ _ _ _ _ _ _ _ _ _ _ _ _ _ _ _ _ _ _ _ _ _ _ _ _ _ _ _ _ _ _ _ _ _ _ _ _ _ _ _ _ _ _ _ _ _ _ _ _ _ _ _ _ _ _ _ _ _ _ _ _ _ _ _ _]
      tunnel: w3933 -> [_ _ _ _ w3985 _ _ _ _ _ _ _ _ _ _ _ _ _ _ _ _ _ _ _ _ _ _ _ _ _ _ _ _ _ _ _ _ _ _ w4217 w4233 w4240 w4248 w4256 w4268 w4276 _ _ _ _ _ _ _ _ _ _ _ _ _ _ _ _ _ _ _ _ _ _ _ _ _ _ _ _ _ _ _ _ _ _ _ _ _ _ _ _ _ _ _ _ _ _ _ _ _ _ _ _ _ _ _ _ _ _ _ _ _ _ _ _ _ _ _ _ _ _ _ _ _ _ _ _ _ _ _ _ _ _ _ _]
      tunnel: w3929 -> [_ _ _ _ w3983 _ _ _ _ _ _ _ _ _ _ _ _ _ _ _ _ _ _ _ _ _ _ _ _ _ _ _ _ _ _ _ _ _ _ _ _ _ _ _ _ _ _ _ _ _ _ _ _ _ _ _ _ _ _ _ _ _ _ _ _ _ _ _ _ _ _ _ _ _ _ _ _ _ _ _ _ _ _ _ _ _ _ _ _ _ _ _ _ _ _ _ _ _ _ _ _ _ _ _ _ _ _ _ _ _ _ _ _ _ _ _ _ _ _ _ _ _ _ w4897 w4907 _ _ _ _ _]
      tunnel: w3927 -> [_ _ _ _ w3979 _ _ _ _ _ _ _ _ _ _ _ _ _ _ _ _ _ _ _ _ _ _ _ _ _ _ _ _ _ _ _ _ _ _ _ _ _ _ _ _ _ _ _ _ _ _ _ _ _ _ _ _ _ _ _ _ _ _ _ _ _ _ _ _ _ _ _ _ _ _ _ _ _ w4555 _ _ _ _ _ w4590 w4601 _ _ _ w4630 _ _ _ _ _ _ _ _ _ _ _ _ _ _ _ _ _ _ _ _ _ _ _ _ _ _ _ _ _ _ _ _ _ _ _ _ _ _ _ _]
      tunnel: w3926 -> [_ _ _ _ _ _ _ _ _ _ _ _ _ _ _ _ _ _ _ _ _ _ _ _ _ _ _ _ _ _ _ _ _ _ _ _ _ _ _ _ _ _ _ _ _ _ _ _ _ _ _ _ _ _ _ _ _ _ _ _ _ _ _ _ _ _ _ _ _ _ _ _ _ _ _ _ _ _ _ _ _ _ _ _ _ _ _ _ w4619 w4629 _ _ _ _ _ _ _ _ _ _ _ _ _ _ _ _ _ _ _ _ _ _ _ _ _ _ _ _ _ _ _ _ _ _ _ _ _ _ _ _]
      tunnel: w3925 -> [_ _ _ _ _ _ _ _ _ _ _ _ _ _ _ _ _ _ _ _ _ _ _ _ _ _ _ _ _ _ _ _ _ _ _ _ _ _ _ _ _ _ _ _ _ _ _ _ _ _ _ _ _ _ _ _ _ _ _ _ _ _ _ _ _ _ _ _ _ _ _ _ _ _ _ _ _ _ _ _ _ _ _ _ _ _ _ _ _ _ _ _ _ _ _ w4674 w4684 w4695 _ _ _ _ _ _ _ _ _ _ _ _ _ _ _ _ _ _ _ _ _ _ _ _ _ _ _ _ _ _ _ _]
      tunnel: w3924 -> [_ _ _ _ _ _ _ _ _ _ _ _ _ _ _ _ _ _ _ _ _ _ _ _ _ _ _ _ _ _ _ _ _ _ _ _ _ _ _ _ _ _ _ _ _ _ _ _ _ _ _ _ _ _ _ _ _ _ _ _ _ _ _ _ _ _ _ _ _ _ _ _ _ _ _ _ _ _ _ _ _ _ _ _ _ _ _ _ _ _ _ _ w4651 _ _ _ _ w4690 _ _ _ _ _ _ _ _ _ _ _ _ _ _ _ _ _ _ _ _ _ _ _ _ _ _ _ _ _ _ _ _]
      tunnel: w3923 -> [_ _ _ _ _ _ _ _ _ _ _ _ _ _ _ _ _ _ _ _ _ _ _ _ _ _ _ _ _ _ _ _ _ _ _ _ _ _ _ _ _ _ _ _ _ _ _ _ _ _ _ _ _ _ _ _ _ _ _ _ _ _ _ _ _ _ _ _ _ _ _ _ _ _ _ _ _ _ _ _ _ _ _ _ _ _ _ _ _ _ _ _ _ _ _ _ _ _ _ _ w4713 w4723 _ _ _ _ _ _ _ _ _ _ _ _ _ _ _ _ _ _ _ _ _ _ _ _ _ _ _ _]
      tunnel: w3922 -> [_ _ _ _ _ _ _ _ _ _ _ _ _ _ _ _ _ _ _ _ _ _ _ _ _ _ _ _ _ _ _ _ _ _ _ _ _ _ _ _ _ _ _ _ _ _ _ _ w4294 w4305 w4313 w4321 w4329 w4337 w4344 w4352 w4360 w4368 _ _ _ _ _ _ _ _ _ _ _ _ _ _ _ _ _ _ _ _ _ _ _ _ _ _ _ _ _ _ _ _ _ _ _ _ _ _ _ _ _ _ _ _ _ _ _ _ _ _ _ _ _ _ _ _ _ _ _ _ _ _ _ _ _ _ _ _ _ _ _ _]
      tunnel: w3921 -> [_ _ _ _ _ _ _ _ _ _ _ _ _ _ w4042 w4053 w4060 w4067 w4074 w4081 w4088 w4095 w4102 w4109 w4116 w4123 w4130 w4137 w4144 w4151 w4158 w4165 w4171 w4177 w4184 w4191 w4198 _ _ _ _ _ _ _ _ _ _ _ _ _ _ _ _ _ _ _ _ _ _ _ _ _ _ _ _ _ _ _ _ _ _ _ _ _ _ _ _ _ _ _ _ _ _ _ _ _ _ _ _ _ _ _ _ _ _ _ _ _ _ _ _ _ _ _ _ _ _ _ _ _ _ _ _ _ _ _ _ _ _ _ _ _ _ _ _ _ _ _ _ _]
      tunnel: w3920 -> [_ _ _ _ _ _ _ _ w4006 w4012 w4018 w4024 _ _ _ _ _ _ _ _ _ _ _ _ _ _ _ _ _ _ _ _ _ _ _ _ _ _ _ _ _ _ _ _ _ _ _ _ _ _ _ _ _ _ _ _ _ _ _ _ _ _ _ _ _ _ _ _ _ _ _ _ _ _ _ _ _ _ _ _ _ _ _ _ _ _ _ _ _ _ _ _ _ _ _ _ _ _ _ _ _ _ _ _ _ _ _ _ _ _ _ _ _ _ _ _ _ _ _ _ _ _ _ _ _ _ _ _ _ _]
      tunnel: w3919 -> [_ _ _ _ _ _ _ _ _ _ _ _ _ _ _ _ _ _ _ _ _ _ _ _ _ _ _ _ _ _ _ _ _ _ _ _ _ _ _ _ _ _ _ _ _ _ _ _ _ _ _ _ _ _ _ _ _ _ _ _ _ _ _ _ _ _ _ _ _ _ _ _ _ _ _ _ _ _ _ _ _ _ _ _ _ _ _ _ _ _ _ _ _ _ _ _ _ _ _ _ _ _ _ _ w4742 w4761 w4763 _ _ _ _ _ _ _ _ _ _ _ _ _ _ _ _ _ _ _ _ _ _ _]
      tunnel: w3918 -> [_ _ _ _ _ _ _ _ _ _ _ _ _ _ _ _ _ _ _ _ _ _ _ _ _ _ _ _ _ _ _ _ _ _ _ _ _ _ _ _ _ _ _ _ _ _ _ _ _ _ _ _ _ _ _ _ _ _ _ _ _ _ _ _ _ _ _ _ _ _ _ _ _ _ _ _ _ _ _ _ _ _ _ _ _ _ _ _ _ _ _ _ _ _ _ _ _ _ _ _ _ _ _ _ _ w4759 _ _ _ w4786 w4796 _ _ _ _ _ _ _ _ _ _ _ _ _ _ _ _ _ _ _]
      tunnel: w3917 -> [_ _ _ _ _ _ _ _ _ _ _ _ _ _ _ _ _ _ _ _ _ _ _ _ _ _ _ _ _ _ _ _ _ _ _ _ _ _ _ _ _ _ _ _ _ _ _ _ _ _ _ _ _ _ _ _ _ _ _ _ _ _ _ _ _ _ _ _ _ _ _ _ _ _ _ _ _ _ w4551 _ _ _ _ _ _ _ _ _ _ _ _ _ _ _ _ _ _ _ _ _ _ _ _ _ _ _ _ _ _ _ _ _ _ _ _ _ _ _ _ _ _ _ _ _ _ _ _ _ _ _]
      tunnel: w3916 -> [_ _ _ _ _ _ _ _ _ _ _ _ _ _ _ _ _ _ _ _ _ _ _ _ _ _ _ _ _ _ _ _ _ _ _ _ _ _ _ _ _ _ _ _ _ _ _ _ _ _ _ _ _ _ _ _ _ _ _ _ _ _ _ _ _ _ _ _ _ _ _ _ _ _ _ _ _ _ _ _ _ _ _ _ _ _ _ _ _ _ _ _ _ _ _ _ _ _ _ _ _ _ _ _ _ _ _ _ _ _ _ _ _ w4821 w4829 _ _ _ _ _ _ _ _ _ _ _ _ _ _ _]
      tunnel: w3915 -> [_ _ _ _ _ _ _ _ _ _ _ _ _ _ _ _ _ _ _ _ _ _ _ _ _ _ _ _ _ _ _ _ _ _ _ _ _ _ _ _ _ _ _ _ _ _ _ _ _ _ _ _ _ _ _ _ _ _ _ _ _ _ _ _ _ _ _ _ _ _ _ _ _ _ _ _ _ _ _ _ _ _ _ _ _ _ _ _ _ _ _ _ _ _ _ _ _ _ _ _ _ _ _ _ _ _ _ _ _ _ _ _ _ _ _ _ _ w4853 w4862 _ _ _ _ _ _ _ _ _ _ _]
      tunnel: w3914 -> [_ _ _ _ _ _ _ _ _ _ _ _ _ _ _ _ _ _ _ _ _ _ _ _ _ _ _ _ _ _ _ _ _ _ _ _ _ _ _ _ _ _ _ _ _ _ _ _ _ _ _ _ _ _ _ _ _ _ _ _ _ _ _ _ _ _ _ _ _ _ w4470 _ _ _ _ _ _ _ _ _ _ _ _ _ _ _ _ _ _ _ _ _ _ _ _ _ _ _ _ _ _ _ _ _ _ _ _ _ _ _ _ _ _ _ _ _ _ _ _ _ _ _ _ _ _ _ _ _ _ _]
      tunnel: w3913 -> [_ _ _ _ _ _ _ _ _ _ _ _ _ _ _ _ _ _ _ _ _ _ _ _ _ _ _ _ _ _ _ _ _ _ _ _ _ _ _ _ _ _ _ _ _ _ _ _ _ _ _ _ _ _ _ _ _ _ _ _ _ w4399 _ _ _ _ _ _ _ _ _ _ _ _ _ _ _ _ _ _ _ _ _ _ _ _ _ _ _ _ _ _ _ _ _ _ _ _ _ _ _ _ _ _ _ _ _ _ _ _ _ _ _ _ _ _ _ _ _ _ _ _ _ _ _ _ _ _ _ _]
      tunnel: w3912 -> [_ _ _ _ _ _ _ _ _ _ _ _ _ _ _ _ _ _ _ _ _ _ _ _ _ _ _ _ _ _ _ _ _ _ _ _ _ _ _ _ _ _ _ _ _ _ _ _ _ _ _ _ _ _ _ _ _ _ _ _ _ _ _ _ w4422 _ _ _ _ _ _ _ _ _ _ _ _ _ _ _ _ _ _ _ _ _ _ _ _ _ _ _ _ _ _ _ _ _ _ _ _ _ _ _ _ _ _ _ _ _ _ _ _ _ _ _ _ _ _ _ _ _ _ _ _ _ _ _ _ _]
      tunnel: w3911 -> [_ _ _ _ _ _ _ _ _ _ _ _ _ _ _ _ _ _ _ _ _ _ _ _ _ _ _ _ _ _ _ _ _ _ _ _ _ _ _ _ _ _ _ _ _ _ _ _ _ _ _ _ _ _ _ _ _ _ _ _ _ _ _ _ _ _ _ w4445 _ _ _ _ _ _ _ _ _ _ _ _ _ _ _ _ _ _ _ _ _ _ _ _ _ _ _ _ _ _ _ _ _ _ _ _ _ _ _ _ _ _ _ _ _ _ _ _ _ _ _ _ _ _ _ _ _ _ _ _ _ _]
      tunnel: w3910 -> [_ _ _ _ _ _ _ _ _ _ _ _ _ _ _ _ _ _ _ _ _ _ _ _ _ _ _ _ _ _ _ _ _ _ _ _ _ _ _ _ _ _ _ _ _ _ _ _ _ _ _ _ _ _ _ _ _ _ _ _ _ _ _ _ _ _ _ _ _ _ _ _ _ _ _ _ _ _ _ _ _ _ _ _ _ _ _ _ _ _ _ _ _ _ _ _ _ _ _ _ _ _ _ _ _ _ _ _ _ _ _ _ _ _ _ _ _ _ _ _ w4874 _ _ _ _ _ _ _ _ _]
      tunnel: w3909 -> [_ _ _ _ _ _ _ _ _ _ _ _ _ _ _ _ _ _ _ _ _ _ _ _ _ _ _ _ _ _ _ _ _ _ _ _ _ _ _ _ _ _ _ _ _ _ _ _ _ _ _ _ _ _ _ _ _ _ _ _ _ _ _ _ _ _ _ _ _ _ _ _ _ _ _ _ _ _ _ _ _ _ _ _ _ _ _ _ _ _ _ _ _ _ _ _ _ _ _ _ _ _ _ _ _ _ _ _ _ _ _ _ _ _ _ _ _ _ _ _ _ _ _ _ _ _ _ w4928 w4938 _]
      frame "---------- Startup ----------" {
        # "Duplicate this frame when creating new messages.  Change this comment in the duplicated frame to describe this message."
        n1587 = Merge Errors(w3951) -> (w3949:errorcluster)
      }
      frame Default {
        # "'Default' case only runs if there is a message that isn't defined in any of the other cases.  Output a programming error."
        n1588 = xnode "Error Ring"("parameter 0"=w3952) -> ("error out"=w3953:errorcluster)
      }
      frame "Initialize" {
        w3964 = TRUE ("Priority Message? (F)")
        # "Initialize - All initialization work should take place in this message, since other loops can potentially enqueue messages that execute immediately after this one."
        n1589 = call-poly "Enqueue Message.vi"("Priority Message? (F)"=w3964, "error in (no error)"=w3969, "Message"="Update_Temp_Limits_UI", "Message Queue"=w3970) -> ("error out"=w3967:errorcluster, "dup Message Queue"=w3965:refnum<queue>)  [unwired: 6 in]
        n1590 = call-poly "Enqueue Message.vi"("Priority Message? (F)"=w3964, "error in (no error)"=w3967, "Message"="Set_Scan_Rate_UI", "Message Queue"=w3965) -> ("error out"=w3966:errorcluster)  [unwired: 6 in, 1 out]
      }
      frame "Error" {
        # "Error - Display an error dialog. This message is sent by the \"Error Handler\" VIs at the end of other loops in this application."
        n1591 = Variant To Data(error in=w3977, type=errorcluster {"status"=FALSE, "code"=0, "source"=""} ("error constant"), Variant=w3975) -> (data=w3973:errorcluster, error out=w3972:errorcluster)
        n1592 = call <vilib>:"Simple Error Handler.vi"("error in (no error)"=w3973) -> ()  [unwired: 4 in, 5 out]
        n1593 = Merge Errors(w3972) -> (w3971:errorcluster)
      }
      frame "Exit" {
        w3980 = TRUE ("Priority Message? (F)")
        w3978 = "Exit" ("Message")
        # "Exit - Exit the application."
        n1594 = Variant To Data(type=errorcluster {"status"=FALSE, "code"=0, "source"=""} ("error constant"), Variant=w3987) -> (data=w3988:errorcluster)  [unwired: 1 in, 1 out]
        n1595 = call <vilib>:"Simple Error Handler.vi"("error in (no error)"=w3988) -> ()  [unwired: 4 in, 5 out]
        n1596 = call "Fire User Event - Stop.vi"("User Event - Stop"=w3992) -> ("error out"=w3991:errorcluster)  [unwired: 10 in]
        n1597 = Release Queue(queue=w3996, error in (no error)=w3990) -> (error out=w3986:errorcluster)  [unwired: 1 in, 2 out]
        n1598 = call-poly "Enqueue Message.vi"("Priority Message? (F)"=w3980, "error in (no error)"=w3986, "Message"=w3978, "Message Queue"=w3985) -> ("error out"=w3984:errorcluster)  [unwired: 6 in, 1 out]
        n1599 = call-poly "Enqueue Message.vi"("Priority Message? (F)"=w3980, "error in (no error)"=w3984, "Message"=w3978, "Message Queue"=w3983) -> ("error out"=w3982:errorcluster)  [unwired: 6 in, 1 out]
        n1600 = call-poly "Enqueue Message.vi"("Priority Message? (F)"=w3980, "error in (no error)"=w3982, "Message"=w3978, "Message Queue"=w3979) -> ("error out"=w3981:errorcluster)  [unwired: 6 in, 1 out]
        n1601 = Merge Errors(w3991, w3981) -> (w3993:errorcluster)
      }
      frame "---------- Process Data ----------" {
        # "Duplicate this frame when creating new messages.  Change this comment in the duplicated frame to describe this message."
        n1602 = Merge Errors(w3999) -> (w3997:errorcluster)
      }
      frame "Process_Data" {
        # "Add density correction for Emerson here."
        # "Duplicate this frame when creating new messages.  Change this comment in the duplicated frame to describe this message."
        n1603 = Unbundle By Name(w4001) -> ("Ritter Data"=→"Ritter Data":T1)
        n1604 = Merge Errors(w4003) -> (w4002:errorcluster)
      }
      frame "---------- Timer Control ----------" {
        # "Place holder, only for organization and readability"
        # "Initialize - All initialization work should take place in this message, since other loops can potentially enqueue messages that execute immediately after this one."
      }
      frame "Reset_TimerA_UI" {
        # "Initialize - All initialization work should take place in this message, since other loops can potentially enqueue messages that execute immediately after this one."
        n1605 = call-poly "Enqueue Message.vi"("Priority Message? (F)"=TRUE, "error in (no error)"=w4011, "Message"="Reset_TimerA", "Message Queue"=w4006) -> ("error out"=w4007:errorcluster)  [unwired: 6 in, 1 out]
      }
      frame "Reset_TimerB_UI" {
        # "Initialize - All initialization work should take place in this message, since other loops can potentially enqueue messages that execute immediately after this one."
        n1606 = call-poly "Enqueue Message.vi"("Priority Message? (F)"=TRUE, "error in (no error)"=w4017, "Message"="Reset_TimerB", "Message Queue"=w4012) -> ("error out"=w4013:errorcluster)  [unwired: 6 in, 1 out]
      }
      frame "Reset_TimerC_UI" {
        # "Initialize - All initialization work should take place in this message, since other loops can potentially enqueue messages that execute immediately after this one."
        n1607 = call-poly "Enqueue Message.vi"("Priority Message? (F)"=TRUE, "error in (no error)"=w4023, "Message"="Reset_TimerC", "Message Queue"=w4018) -> ("error out"=w4019:errorcluster)  [unwired: 6 in, 1 out]
      }
      frame "Reset_TimerD_UI" {
        # "Initialize - All initialization work should take place in this message, since other loops can potentially enqueue messages that execute immediately after this one."
        n1608 = call-poly "Enqueue Message.vi"("Priority Message? (F)"=TRUE, "error in (no error)"=w4029, "Message"="Reset_TimerD", "Message Queue"=w4024) -> ("error out"=w4025:errorcluster)  [unwired: 6 in, 1 out]
      }
      frame "DisplayValuesFromTimer" {
        # "Initialize - All initialization work should take place in this message, since other loops can potentially enqueue messages that execute immediately after this one."
        n1609 = Variant To Data(error in=w4039, type=T68 {"Station A-Timer"=[], "Station B-Timer"=[], "Station C-Timer"=[], "Station D-Timer"=[], "Timer A"=0.0, "Timer B"=0.0, "Timer C"=0.0, "Timer D"=0.0, "TimerA (String)"="", "TimerB (String)"="", "TimerC (String)"="", "TimerD (String)"="", "TimerA (H:M:S)"="", "TimerB (H:M:S)"="", "TimerC (H:M:S)"="", "TimerD (H:M:S)"=""} ("Timer"), Variant=w4038) -> (data=w4034:T68, error out=w4032:errorcluster)
        n1610 = Bundle By Name(cluster=w4036, "Timer Data"=w4034) -> (w4035:T67)
        n1611 = call-poly "Enqueue Message.vi"("error in (no error)"=w4032, "Message"="Process_Data", "Message Queue"=w4030) -> ("error out"=w4031:errorcluster)  [unwired: 7 in, 1 out]
      }
      frame "---------- MW100 Control ----------" {
        # "Place holder, only for organization and readability"
        # "Initialize - All initialization work should take place in this message, since other loops can potentially enqueue messages that execute immediately after this one."
      }
      frame "Set_MW100_VISA_Name_UI" {
        n1612 = Variant To Data(error in=w4048, type="", Variant=w4046) -> (data=w4043:string, error out=w4047:errorcluster)
        n1613 = call-poly "Enqueue Message.vi"("Priority Message? (F)"=TRUE, "error in (no error)"=w4047, "Message Data"=w4043, "Message"="Set_MW100_VISA_Name", "Message Queue"=w4042) -> ("error out"=w4045:errorcluster)  [unwired: 5 in, 1 out]
      }
      frame "MainPower_MW100_UI" {
        n1614 = call-poly "Enqueue Message.vi"("Priority Message? (F)"=TRUE, "error in (no error)"=w4058, "Message Data"="Main Power", "Message"="MainPower_MW100", "Message Queue"=w4053) -> ("error out"=w4054:errorcluster)  [unwired: 5 in, 1 out]
      }
      frame "Set_Valves_StationA_MW100_UI" {
        n1615 = call-poly "Enqueue Message.vi"("Priority Message? (F)"=TRUE, "error in (no error)"=w4065, "Message Data"="Station A Valve Setting", "Message"="Set_Valves_StationA_MW100", "Message Queue"=w4060) -> ("error out"=w4061:errorcluster)  [unwired: 5 in, 1 out]
      }
      frame "Set_Valves_StationB_MW100_UI" {
        n1616 = call-poly "Enqueue Message.vi"("Priority Message? (F)"=TRUE, "error in (no error)"=w4072, "Message Data"="Station B Valve Setting", "Message"="Set_Valves_StationB_MW100", "Message Queue"=w4067) -> ("error out"=w4068:errorcluster)  [unwired: 5 in, 1 out]
      }
      frame "Set_Valves_StationC_MW100_UI" {
        n1617 = call-poly "Enqueue Message.vi"("Priority Message? (F)"=TRUE, "error in (no error)"=w4079, "Message Data"="Station C Valve Setting", "Message"="Set_Valves_StationC_MW100", "Message Queue"=w4074) -> ("error out"=w4075:errorcluster)  [unwired: 5 in, 1 out]
      }
      frame "Set_Valves_StationD_MW100_UI" {
        n1618 = call-poly "Enqueue Message.vi"("Priority Message? (F)"=TRUE, "error in (no error)"=w4086, "Message Data"="Station D Valve Setting", "Message"="Set_Valves_StationD_MW100", "Message Queue"=w4081) -> ("error out"=w4082:errorcluster)  [unwired: 5 in, 1 out]
      }
      frame "Inlet_Valve_A_MW100_UI" {
        n1619 = call-poly "Enqueue Message.vi"("Priority Message? (F)"=TRUE, "error in (no error)"=w4093, "Message Data"="Inlet Valve A", "Message"="Inlet_Valve_A_MW100", "Message Queue"=w4088) -> ("error out"=w4089:errorcluster)  [unwired: 5 in, 1 out]
      }
      frame "Inlet_Valve_B_MW100_UI" {
        n1620 = call-poly "Enqueue Message.vi"("Priority Message? (F)"=TRUE, "error in (no error)"=w4100, "Message Data"="Inlet Valve B", "Message"="Inlet_Valve_B_MW100", "Message Queue"=w4095) -> ("error out"=w4096:errorcluster)  [unwired: 5 in, 1 out]
      }
      frame "Inlet_Valve_C_MW100_UI" {
        n1621 = call-poly "Enqueue Message.vi"("Priority Message? (F)"=TRUE, "error in (no error)"=w4107, "Message Data"="Inlet Valve C", "Message"="Inlet_Valve_C_MW100", "Message Queue"=w4102) -> ("error out"=w4103:errorcluster)  [unwired: 5 in, 1 out]
      }
      frame "Inlet_Valve_D_MW100_UI" {
        n1622 = call-poly "Enqueue Message.vi"("Priority Message? (F)"=TRUE, "error in (no error)"=w4114, "Message Data"="Inlet Valve D", "Message"="Inlet_Valve_D_MW100", "Message Queue"=w4109) -> ("error out"=w4110:errorcluster)  [unwired: 5 in, 1 out]
      }
      frame "Drain_Valve_A_MW100_UI" {
        n1623 = call-poly "Enqueue Message.vi"("Priority Message? (F)"=TRUE, "error in (no error)"=w4121, "Message Data"="Drain Valve A", "Message"="Drain_Valve_A_MW100", "Message Queue"=w4116) -> ("error out"=w4117:errorcluster)  [unwired: 5 in, 1 out]
      }
      frame "Drain_Valve_B_MW100_UI" {
        n1624 = call-poly "Enqueue Message.vi"("Priority Message? (F)"=TRUE, "error in (no error)"=w4128, "Message Data"="Drain Valve B", "Message"="Drain_Valve_B_MW100", "Message Queue"=w4123) -> ("error out"=w4124:errorcluster)  [unwired: 5 in, 1 out]
      }
      frame "Drain_Valve_C_MW100_UI" {
        n1625 = call-poly "Enqueue Message.vi"("Priority Message? (F)"=TRUE, "error in (no error)"=w4135, "Message Data"="Drain Valve C", "Message"="Drain_Valve_C_MW100", "Message Queue"=w4130) -> ("error out"=w4131:errorcluster)  [unwired: 5 in, 1 out]
      }
      frame "Drain_Valve_D_MW100_UI" {
        n1626 = call-poly "Enqueue Message.vi"("Priority Message? (F)"=TRUE, "error in (no error)"=w4142, "Message Data"="Drain Valve D", "Message"="Drain_Valve_D_MW100", "Message Queue"=w4137) -> ("error out"=w4138:errorcluster)  [unwired: 5 in, 1 out]
      }
      frame "Outlet_Valve_A_MW100_UI" {
        n1627 = call-poly "Enqueue Message.vi"("Priority Message? (F)"=TRUE, "error in (no error)"=w4149, "Message Data"="Outlet Valve A", "Message"="Outlet_Valve_A_MW100", "Message Queue"=w4144) -> ("error out"=w4145:errorcluster)  [unwired: 5 in, 1 out]
      }
      frame "Outlet_Valve_B_MW100_UI" {
        n1628 = call-poly "Enqueue Message.vi"("Priority Message? (F)"=TRUE, "error in (no error)"=w4156, "Message Data"="Outlet Valve B", "Message"="Outlet_Valve_B_MW100", "Message Queue"=w4151) -> ("error out"=w4152:errorcluster)  [unwired: 5 in, 1 out]
      }
      frame "Outlet_Valve_C_MW100_UI" {
        n1629 = call-poly "Enqueue Message.vi"("Priority Message? (F)"=TRUE, "error in (no error)"=w4163, "Message Data"="Outlet Valve C", "Message"="Outlet_Valve_C_MW100", "Message Queue"=w4158) -> ("error out"=w4159:errorcluster)  [unwired: 5 in, 1 out]
      }
      frame "Outlet_Valve_D_MW100_UI" {
        n1630 = call-poly "Enqueue Message.vi"("Priority Message? (F)"=TRUE, "error in (no error)"=w4170, "Message Data"="Outlet Valve D", "Message"="Outlet_Valve_D_MW100", "Message Queue"=w4165) -> ("error out"=w4166:errorcluster)  [unwired: 5 in, 1 out]
      }
      frame "Start_Intellifaucet_MW100_UI" {
        n1631 = call-poly "Enqueue Message.vi"("Priority Message? (F)"=TRUE, "error in (no error)"=w4176, "Message"="Start_Intellifaucet_MW100", "Message Queue"=w4171) -> ("error out"=w4172:errorcluster)  [unwired: 6 in, 1 out]
      }
      frame "Stop_Intellifaucet_MW100_UI" {
        n1632 = call-poly "Enqueue Message.vi"("Priority Message? (F)"=TRUE, "error in (no error)"=w4182, "Message"="Stop_Intellifaucet_MW100", "Message Queue"=w4177) -> ("error out"=w4178:errorcluster)  [unwired: 6 in, 1 out]
      }
      frame "Adjust_Temp_Intellifaucet_MW100_UI" {
